vi "measurementGlobal.vi"() -> ()   [LabVIEW 2017]
uses:
  Controls/saveDataOption.ctl
  Controls/postProData.ctl
  Controls/chanType.ctl
  Controls/U.ctl
  Controls/chan&Span.ctl
  Controls/chanData.ctl
  Controls/blocksWTInfo.ctl
panel:
  in  "Tab Control":T1(tab)
  in  "Measurement No.":i32
  in  "Data Acquisition":T2(ring)
  in  "Setup":u16(ring) items=["Run Programme", "Show Setup"]
  in  "Sampling Period (s)":dbl
  in  "Output No of samples":i32
  in  "Acquisition-Plug-In.vi":string(combo)
  in  "Block Index":i32
  in  "Input No of Blocks":i32
  in  "Input No of samples":i32
  in  "Input Sampling rate (Hz)":dbl
  in  "Actual Measurement time (mins)":dbl
  in  "Average time (mins)":dbl
  in  "New Data Post-Pro Folder":bool
  in  "Post-Pro Folder Name":path
  in  "Folder Name":string
  in  "New Measurement Folder":bool
  out "Comments":string
  in  "Folder Path":path
  in  "Save Data Option":T3
  in  "WT Information":dbl[](array[numeric])
  in  "Chan + Span Limit":T4[](array[typedef]) {"input terminal configuration" items=["Default"=-1, "RSE"=10083, "NRSE"=10078, "Differential"=10106, "Pseudodifferential"=12529]}
  out "error out":errorcluster
  in  "Analogue Data (volts)":dbl[][](array[numeric])
  out "taskReadInputs":refnum<k21>
  in  "Device Name":string
  in  "Non-Uniform Data Output":T5[](array[typedef])
  in  "Non-Uniform Data":T5[](array[typedef])
  in  "Signal Processing Type":T6[](array[typedef])
  in  "Number of PP Channels":i32[](array[numeric])
  in  "PostProData":T7[](array[typedef])
  in  "PostProDataPerBlock":T7[][](array[typedef])
  in  "WT Info.":T8
  in  "Accum. U":T9[](array[typedef])
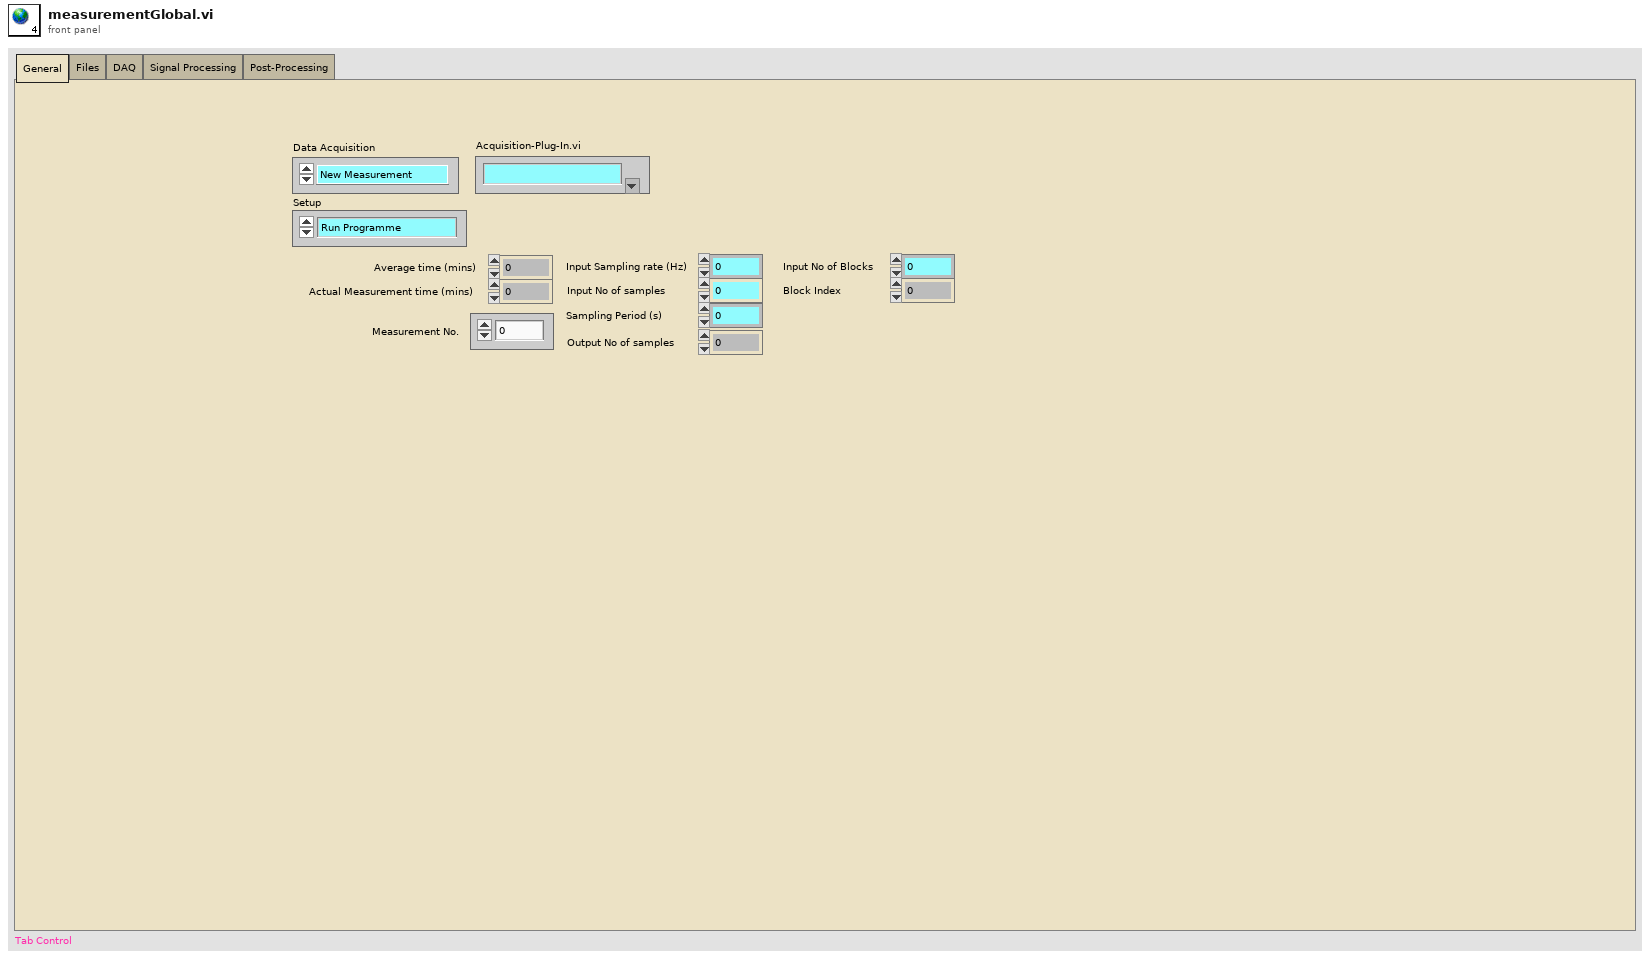
[diagram p1: front panel]
types:
  T1 = enum32{"General", "Files", "DAQ", "Signal Processing", "Post-Processing"}
  T2 = enum16{"New Measurement", "Post-process Raw Data"}
  T3 = typedef "saveDataOption.ctl" = enum16{"Save Data", "Do Not Save Data"}
  T4 = typedef "chan&Span.ctl" = cluster{"Chan No.":i32, "Low Volt Limit (-10V)":dbl, "High Volt Limit (10V)":dbl, "input terminal configuration":i32}
  T5 = typedef "chanData.ctl" = cluster{"Raw Data":dbl[], "Channel Name":string}
  T6 = typedef "chanType.ctl" = enum16{"Default", "Chell 64-Channel"}
  T7 = typedef "postProData.ctl" = cluster{"Channel":string, "Samples":i32, "U":dbl, "u^2":dbl, "u^3":dbl, "u^4":dbl, "Kurtosis":dbl, "Skewness":dbl, "Turb":dbl}
  T8 = typedef "blocksWTInfo.ctl" = cluster{"Velocity (ms^-1)":dbl, "Density (kgm^-3)":dbl, "Pressure (Pa)":dbl, "Temperature (C)":dbl}
  T9 = typedef "U.ctl" = cluster{"Samples":dbl, "U":dbl, "U2":dbl, "U3":dbl, "U4":dbl}
diagram:
